vi "Autonomous Independent.vi"() -> ()   [LabVIEW 2013]
doc: "This VI is called when autonomous begins, and will automatically be terminated when autonomous ends. You can carry out timed or sensor driven robot movement independently without needing to return to the caller."
uses:
  Begin/Global Variables.vi
  Begin/Global Refnums.vi
panel:
  out "Index 2":i32
  # "Be sure to right-click and choose Data Operations>>Make Current Value default if you want to save the array values with the VI"
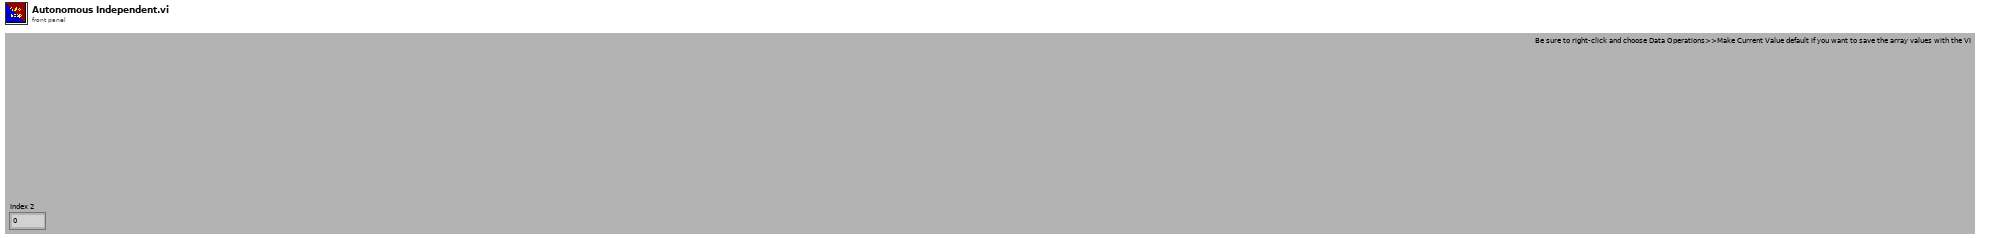
[diagram p1: front panel]
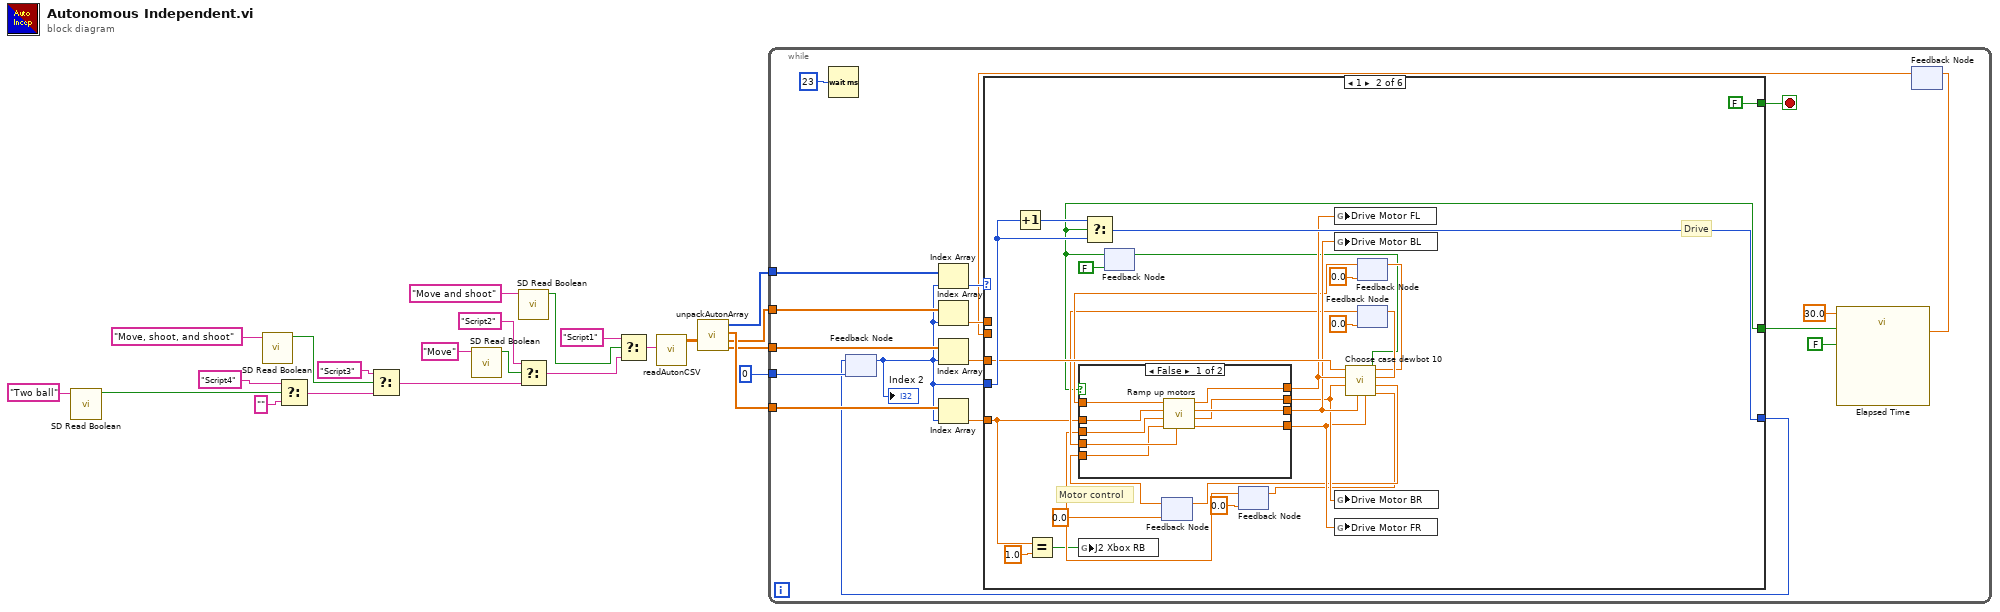
[diagram p0: block diagram]
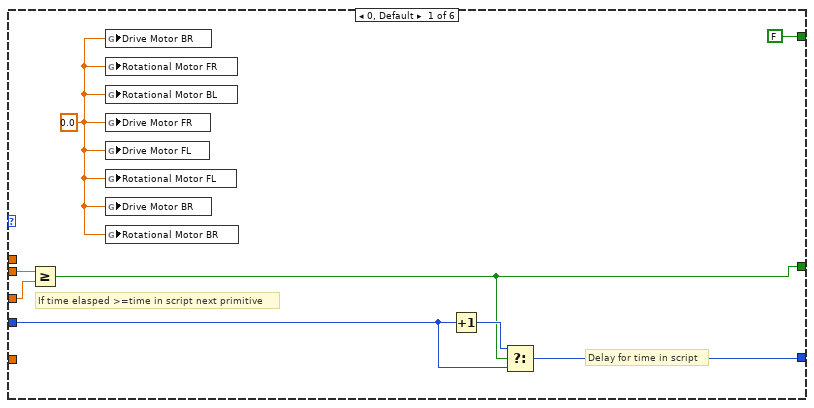
[diagram p2: hidden frame]
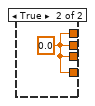
[diagram p3: hidden frame]
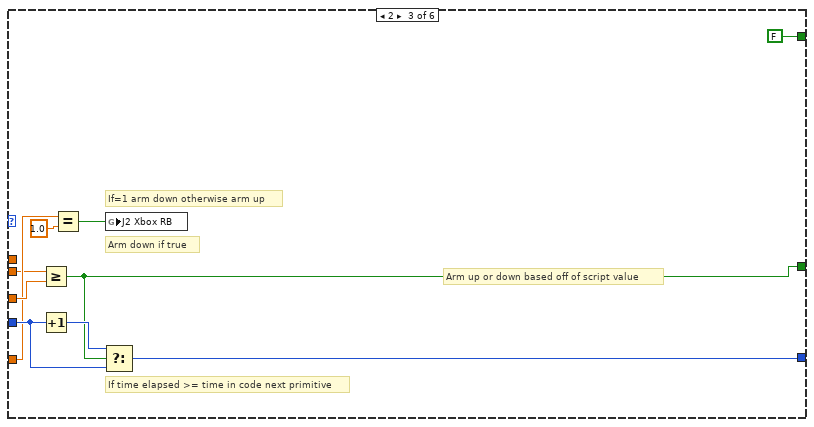
[diagram p4: hidden frame]
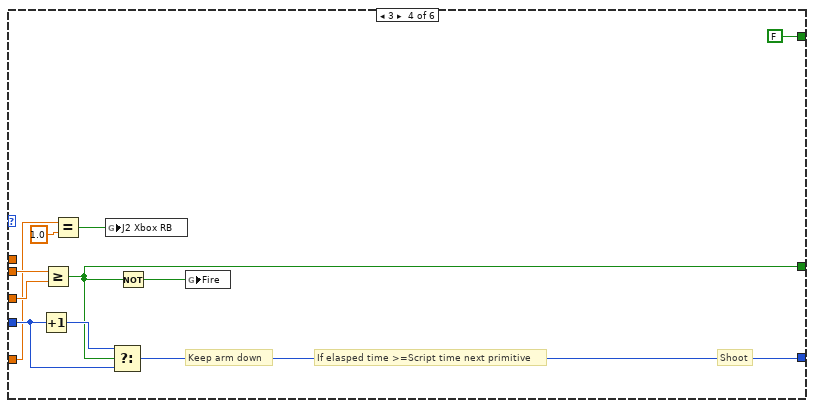
[diagram p5: hidden frame]
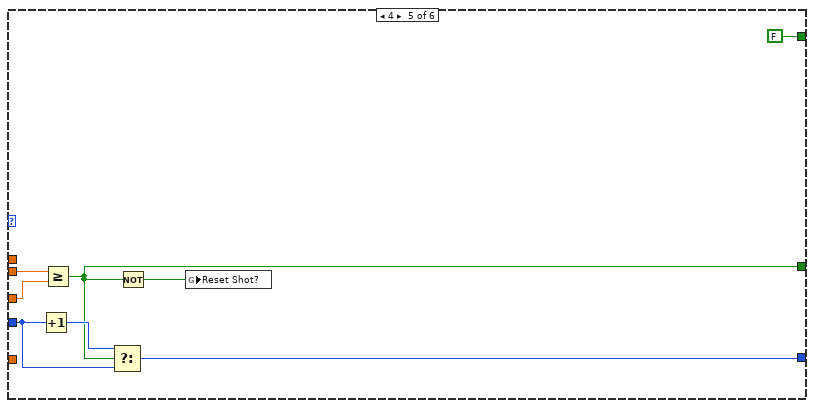
[diagram p6: hidden frame]
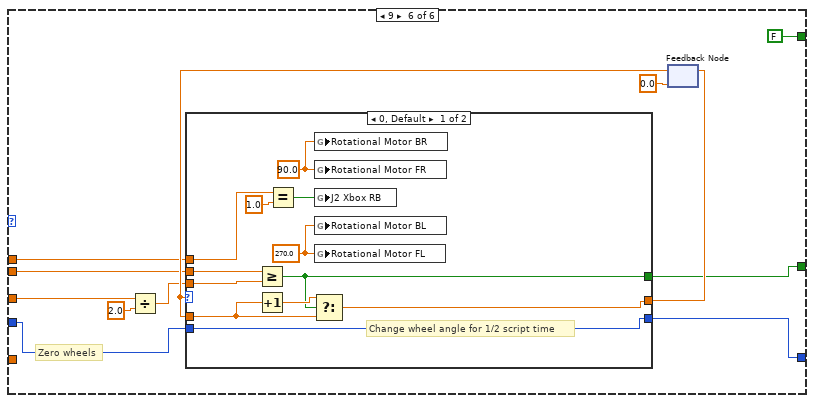
[diagram p7: hidden frame]
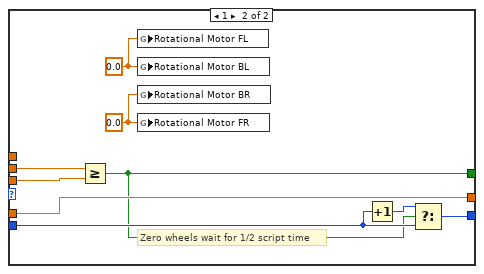
[diagram p8: hidden frame]
diagram:
  n1 = call <vilib>:"SD Read Boolean.vi"("Name"="Two ball") -> ("Boolean"=w3:bool)  [unwired: 8 in, 2 out]
  n2 = call <vilib>:"SD Read Boolean.vi"("Name"="Move, shoot, and shoot") -> ("Boolean"=w9:bool)  [unwired: 8 in, 2 out]
  n3 = Select(t="Script4" ("Name"), s=w3, f="" ("Name")) -> (s? t:f=w1:string)
  n4 = Select(t="Script3" ("Name"), s=w9, f=w1) -> (s? t:f=w7:string)
  n5 = call <vilib>:"SD Read Boolean.vi"("Name"="Move") -> ("Boolean"=w14:bool)  [unwired: 8 in, 2 out]
  n6 = call <vilib>:"SD Read Boolean.vi"("Name"="Move and shoot") -> ("Boolean"=w12:bool)  [unwired: 8 in, 2 out]
  n7 = Select(t="Script2" ("Name"), s=w14, f=w7) -> (s? t:f=w13:string)
  n8 = Select(t="Script1" ("Name"), s=w12, f=w13) -> (s? t:f=w17:string)
  n9 = call "readAutonCSV.vi"("AutonFile"=w17) -> ("AutonArray"=w23:dbl[][])  [unwired: 7 in]
  n10 = call "unpackAutonArray.vi"("all rows"=w23) -> ("Distance/time"=w18:dbl[], "Heading/Shoot angle"=w19:dbl[], "Power/Arm"=w20:dbl[], "Primitive"=w21:i16[])  [unwired: 6 in, 1 out]
  n11 = while {
    tunnel: w21 -> [w38]
    tunnel: w20 -> [w37]
    tunnel: w19 -> [w36]
    tunnel: w18 -> [w35]
    tunnel: 0 -> [w33]
    stop <- w39 stop-if-true
    n12 = Wait (ms)(milliseconds to wait=u32 23) -> ()  [unwired: 1 out]
    n13 = feedback #1(w33) -> (w34:i32)
    "Index 2" <- w34
    n14 = Index Array(array=w38, index=w34) -> (element=w41:i16)
    n15 = Index Array(array=w36, index=w34) -> (element=w29:dbl)
    n16 = Index Array(array=w35, index=w34) -> (element=w31:dbl)
    n17 = Index Array(array=w37, index=w34) -> (element=w30:dbl)
    n18 = feedback #2() -> (w26:dbl)  [unwired: 1 in]
    n19 = case shown="1" w41 {
      tunnel: w29 -> [_ _ _ _ _ w122]
      tunnel: w30 -> [_ w51 w88 w99 _ _]
      tunnel: [w48 w75 w93 w105 w113 w124] -> w32
      tunnel: w31 -> [w45 w73 w92 w103 w111 w120]
      tunnel: [FALSE ("Next primitive?") FALSE ("Next primitive?") FALSE ("Next primitive?") FALSE ("Next primitive?") FALSE ("Next primitive?") FALSE ("Next primitive?")] -> w39
      tunnel: w34 -> [w47 w74 w94 w107 w114 w125]
      tunnel: [w44 w55 w90 w101 w108 w121] -> w28
      tunnel: w26 -> [w46 _ w87 w102 w110 w117]
      frame 0, Default {
        w43 = 0.0
        # "Delay for time in script"
        # "If time elasped >=time in script next primitive"
        n20 = Greater Or Equal?(x=w46, y=w45) -> (x >= y?=w44:bool)
        n21 = global write "Global Variables.vi" "Drive Motor BR"(w43) -> ()
        n22 = global write "Global Variables.vi" "Rotational Motor FR"(w43) -> ()
        n23 = global write "Global Variables.vi" "Rotational Motor BL"(w43) -> ()
        n24 = global write "Global Variables.vi" "Drive Motor FR"(w43) -> ()
        n25 = global write "Global Variables.vi" "Drive Motor FL"(w43) -> ()
        n26 = global write "Global Variables.vi" "Rotational Motor FL"(w43) -> ()
        n27 = global write "Global Variables.vi" "Drive Motor BR"(w43) -> ()
        n28 = global write "Global Variables.vi" "Rotational Motor BR"(w43) -> ()
        n29 = Increment(x=w47) -> (x+1=w49:i32)
        n30 = Select(t=w49, s=w44, f=w47) -> (s? t:f=w48:i32)
      }
      frame 1 {
        # "Motor control"
        # "Drive"
        n31 = Increment(x=w74) -> (x+1=w76:i32)
        n32 = Equal?(x=w51, y=1.0) -> (x = y?=w52:bool)
        n33 = global write "Global Variables.vi" "J2 Xbox RB"(w52) -> ()
        n34 = feedback #3(FALSE ("Next primitive?")) -> (w55:bool)
        n35 = Select(t=w76, s=w55, f=w74) -> (s? t:f=w75:i32)
        n36 = feedback #4(0.0 ("Last BL motor value")) -> (w64:dbl)
        n37 = feedback #5(0.0 ("Last FR motor value")) -> (w62:dbl)
        n38 = feedback #6(0.0 ("Last FL motor value")) -> (w68:dbl)
        n39 = feedback #7(0.0 ("Last BR motor value")) -> (w66:dbl)
        n40 = case shown="False" w55 {
          tunnel: w51 -> [w85 _]
          tunnel: [w84 w86] -> w72
          tunnel: [w83 w86] -> w71
          tunnel: [w82 w86] -> w70
          tunnel: [w81 w86] -> w69
          tunnel: w68 -> [w80 _]
          tunnel: w66 -> [w79 _]
          tunnel: w64 -> [w78 _]
          tunnel: w62 -> [w77 _]
          frame False {
            n41 = call "Ramp up motors.vi"("Last BR motor value"=w79, "Last BL motor value"=w78, "Last FR motor value"=w77, "Set motor value"=w85, "Last FL motor value"=w80) -> ("Next FR motor value"=w81:dbl, "Next BR motor value"=w82:dbl, "Next BL motor value"=w83:dbl, "Next FL motor value"=w84:dbl)  [unwired: 3 in]
          }
          frame True {
            w86 = 0.0 ("Next FL motor value")
          }
        }
        n42 = global write "Global Variables.vi" "Drive Motor FL"(w72) -> ()
        n43 = global write "Global Variables.vi" "Drive Motor BL"(w71) -> ()
        n44 = global write "Global Variables.vi" "Drive Motor BR"(w70) -> ()
        n45 = global write "Global Variables.vi" "Drive Motor FR"(w69) -> ()
        n46 = call "Choose case dewbot 10.vi"("Next FR motor value"=w69, "Next BL motor value"=w71, "Next BR motor value"=w70, "Next FL motor value"=w72, "Set Tac value"=w73) -> ("Last FR motor value"=w63:dbl, "Last BL motor value"=w65:dbl, "Last BR motor value"=w67:dbl, "Last FL motor value"=w57:dbl, "Next primitive?"=w56:bool)  [unwired: 2 in]
        n47 = feedback-in #3(w56) -> ()
        n48 = feedback-in #4(w65) -> ()
        n49 = feedback-in #5(w63) -> ()
        n50 = feedback-in #6(w57) -> ()
        n51 = feedback-in #7(w67) -> ()
      }
      frame 2 {
        # "Arm down if true"
        # "If time elapsed >= time in code next primitive"
        # "If=1 arm down otherwise arm up"
        # "Arm up or down based off of script value"
        n52 = Greater Or Equal?(x=w87, y=w92) -> (x >= y?=w90:bool)
        n53 = Increment(x=w94) -> (x+1=w95:i32)
        n54 = Equal?(x=w88, y=1.0) -> (x = y?=w89:bool)
        n55 = Select(t=w95, s=w90, f=w94) -> (s? t:f=w93:i32)
        n56 = global write "Global Variables.vi" "J2 Xbox RB"(w89) -> ()
      }
      frame 3 {
        # "Keep arm down"
        # "If elasped time >=Script time next primitive"
        # "Shoot"
        n57 = Increment(x=w107) -> (x+1=w106:i32)
        n58 = Greater Or Equal?(x=w102, y=w103) -> (x >= y?=w101:bool)
        n59 = Equal?(x=w99, y=1.0) -> (x = y?=w97:bool)
        n60 = global write "Global Variables.vi" "J2 Xbox RB"(w97) -> ()
        n61 = Select(t=w106, s=w101, f=w107) -> (s? t:f=w105:i32)
        n62 = Not(x=w101) -> (.not. x?=w104:bool)
        n63 = global write "Global Refnums.vi" "Fire"(w104) -> ()
      }
      frame 4 {
        n64 = Increment(x=w114) -> (x+1=w115:i32)
        n65 = Greater Or Equal?(x=w110, y=w111) -> (x >= y?=w108:bool)
        n66 = Select(t=w115, s=w108, f=w114) -> (s? t:f=w113:i32)
        n67 = Not(x=w108) -> (.not. x?=w109:bool)
        n68 = global write "Global Refnums.vi" "Reset Shot?"(w109) -> ()
      }
      frame 9 {
        # "Zero wheels"
        n69 = Divide(x=w120, y=2.0) -> (x/y=w119:dbl)
        n70 = feedback #8(0.0) -> (w126:dbl)
        n71 = case shown="0, Default" w126 {
          tunnel: [w131 w143] -> w127
          tunnel: w126 -> [w132 w143]
          tunnel: w125 -> [w134 w144]
          tunnel: [w134 w145] -> w124
          tunnel: w122 -> [w135 _]
          tunnel: w119 -> [w129 w141]
          tunnel: [w130 w142] -> w121
          tunnel: w117 -> [w128 w140]
          frame 0, Default {
            w137 = 270.0 ("Rotational Motor FL")
            w136 = 90.0 ("Rotational Motor FR")
            # "Change wheel angle for 1/2 script time"
            n72 = Greater Or Equal?(x=w128, y=w129) -> (x >= y?=w130:bool)
            n73 = Increment(x=w132) -> (x+1=w133:dbl)
            n74 = Equal?(x=w135, y=1.0) -> (x = y?=w139:bool)
            n75 = Select(t=w133, s=w130, f=w132) -> (s? t:f=w131:dbl)
            n76 = global write "Global Variables.vi" "Rotational Motor BR"(w136) -> ()
            n77 = global write "Global Variables.vi" "Rotational Motor FR"(w136) -> ()
            n78 = global write "Global Variables.vi" "J2 Xbox RB"(w139) -> ()
            n79 = global write "Global Variables.vi" "Rotational Motor BL"(w137) -> ()
            n80 = global write "Global Variables.vi" "Rotational Motor FL"(w137) -> ()
          }
          frame 1 {
            w148 = 0.0 ("Rotational Motor BL")
            w147 = 0.0
            # "Zero wheels wait for 1/2 script time"
            n81 = Greater Or Equal?(x=w140, y=w141) -> (x >= y?=w142:bool)
            n82 = global write "Global Variables.vi" "Rotational Motor FL"(w148) -> ()
            n83 = global write "Global Variables.vi" "Rotational Motor BL"(w148) -> ()
            n84 = global write "Global Variables.vi" "Rotational Motor BR"(w147) -> ()
            n85 = global write "Global Variables.vi" "Rotational Motor FR"(w147) -> ()
            n86 = Increment(x=w144) -> (x+1=w146:i32)
            n87 = Select(t=w146, s=w142, f=w144) -> (s? t:f=w145:i32)
          }
        }
        n88 = feedback-in #8(w127) -> ()
      }
    }
    n89 = feedback-in #1(w32) -> ()
    n90 = call "Elapsed Time"("Time Target (s)"=30.0, "Reset"=w28, "Auto Reset"=FALSE) -> ("Elapsed Time (s)"=w24:dbl)  [unwired: 9 in, 7 out]
    n91 = feedback-in #2(w24) -> ()
  }
